vi "String to SingleComplex (Scalar).vi"(10 "Value (String)":string) -> (1 "Rest of string":string, 2 "Value (CSG)":csg, 3 "offset past number":i32)   [LabVIEW 2013, in "OpenScalar.lvlib"]
uses:
  OpenScalar.lvlib
  Get Decimal Separator.vi
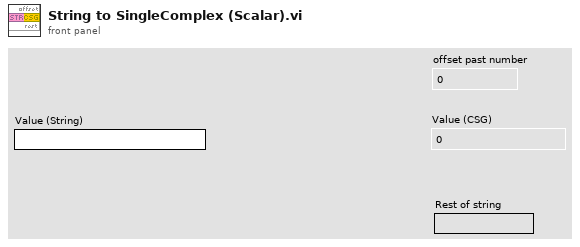
[diagram p1: front panel]
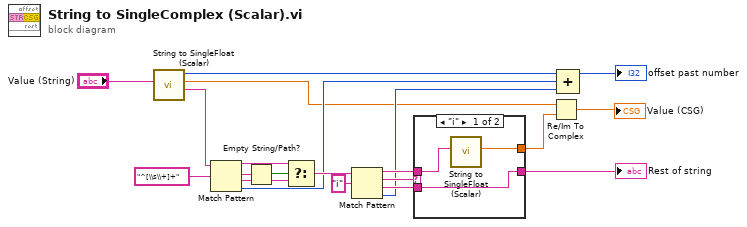
[diagram p0: block diagram]
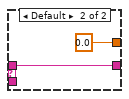
[diagram p2: hidden frame]
diagram:
  n1 = call "String to SingleFloat (Scalar).vi"("Value (String)"="Value (String)") -> ("Rest of string"=w4:string, "Value (Single)"=w5:sgl, "offset past number"=w6:i32)  [unwired: 8 in]
  n2 = Match Pattern(string=w4, regular expression="^[\\s\\+]+") -> (before substring=w12:string, match substring=w14:string, after substring=w11:string, offset past match=w8:i32)  [unwired: 1 in]
  n3 = Empty String/Path?(string/path=w14) -> (empty?=w13:bool)
  n4 = Select(t=w12, s=w13, f=w11) -> (s? t:f=w10:string)
  n5 = Match Pattern(string=w10, regular expression="i") -> (before substring=w17:string, match substring=w19:string, after substring=w16:string, offset past match=w9:i32)  [unwired: 1 in]
  n6 = case shown="\"i\"" w19 {
    tunnel: [w22 sgl 0.0 ("y")] -> w18
    tunnel: w17 -> [w21 w24]
    tunnel: [w23 w24] -> w3
    tunnel: w16 -> [w23 _]
    frame "i" {
      n7 = call "String to SingleFloat (Scalar).vi"("Value (String)"=w21) -> ("Value (Single)"=w22:sgl)  [unwired: 8 in, 2 out]
    }
    frame Default {
    }
  }
  "Rest of string" <- w3
  n8 = Re/Im To Complex(1:w18, 2:w5) -> (0:→"Value (CSG)":csg)
  n9 = Compound Arithmetic op=ADD(w6, w8, w9) -> (→"offset past number":i32)
